vi "SubVI_StaticCharasteristic_YL.vi"(5 "Xs":dbl, 6 "U":dbl[](array[numeric]), 7 "Kvs":dbl, 8 "Kvc":dbl, 9 "Qe":dbl, 10 "rho":dbl, 11 "KL":dbl) -> (1 "Cluster":cluster{"U":dbl[], "YL":dbl[]})   [LabVIEW 2020]
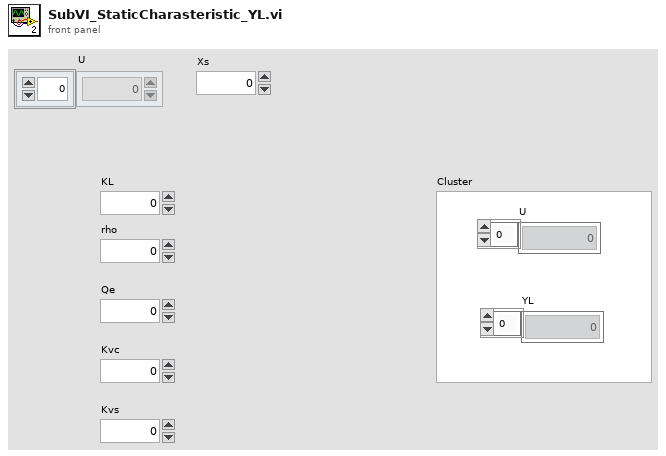
[diagram p1: front panel]
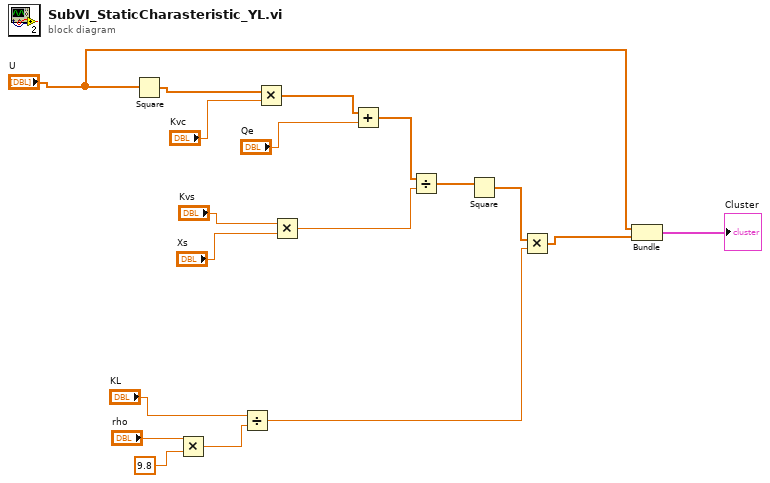
[diagram p0: block diagram]
diagram:
  n1 = Square(x="U") -> (x^2=w14:dbl[])
  n2 = Multiply(x="rho", y=9.8) -> (x*y=w15:dbl)
  n3 = Divide(x="KL", y=w15) -> (x/y=w4:dbl)
  n4 = Multiply(x=w14, y="Kvc") -> (x*y=w12:dbl[])
  n5 = Multiply(x="Kvs", y="Xs") -> (x*y=w7:dbl)
  n6 = Add(x=w12, y="Qe") -> (x+y=w8:dbl[])
  n7 = Divide(x=w8, y=w7) -> (x/y=w6:dbl[])
  n8 = Square(x=w6) -> (x^2=w5:dbl[])
  n9 = Multiply(x=w5, y=w4) -> (x*y=w2:dbl[])
  n10 = Bundle("U"="U", w2) -> (→"Cluster":cluster{"U":dbl[], dbl[]})  [unwired: 1 in]
